vi "daq_board__V3 (2).vi"() -> ()   [LabVIEW 2014]
uses:
  <vilib>/express/express arith-compare/Formula/XNode/ExpressFormulaBlockNode.xnode
  <vilib>/express/express shared/transition.llb/Dynamic To Waveform Array.vi
  <vilib>/express/express arith-compare/Formula/Block/exnFormulaBlock how many pts in the wave.vi
  <vilib>/express/express shared/ex_Modify Signal Name.vi
  <vilib>/express/express shared/transition.llb/Waveform Array To Dynamic.vi
  <vilib>/gmath/NI_Gmath.lvlib
  <vilib>/Utility/file.llb/Write To Spreadsheet File (DBL).vi
  <vilib>/event_ctls.llb/eventsource.ctl
panel:
  out "OK":bool
  in  "Enable":bool=TRUE
  in  "Numeric":i32
  out "Time":u32
  out "true":bool
  in  "stop":bool
  out "time passed (seconds)":i32
  out "Pressure(Torr)":dbl
  out "Voltage(V)":dbl
  out "Waveform Chart 2":dynamicdata(graph)
  out "F-format string":string
  in  "Time to wait(in sec)":dbl
  out "concatenated string":string
  out "Waveform Chart":dbl[](graph)
  in  "stop (F)":bool
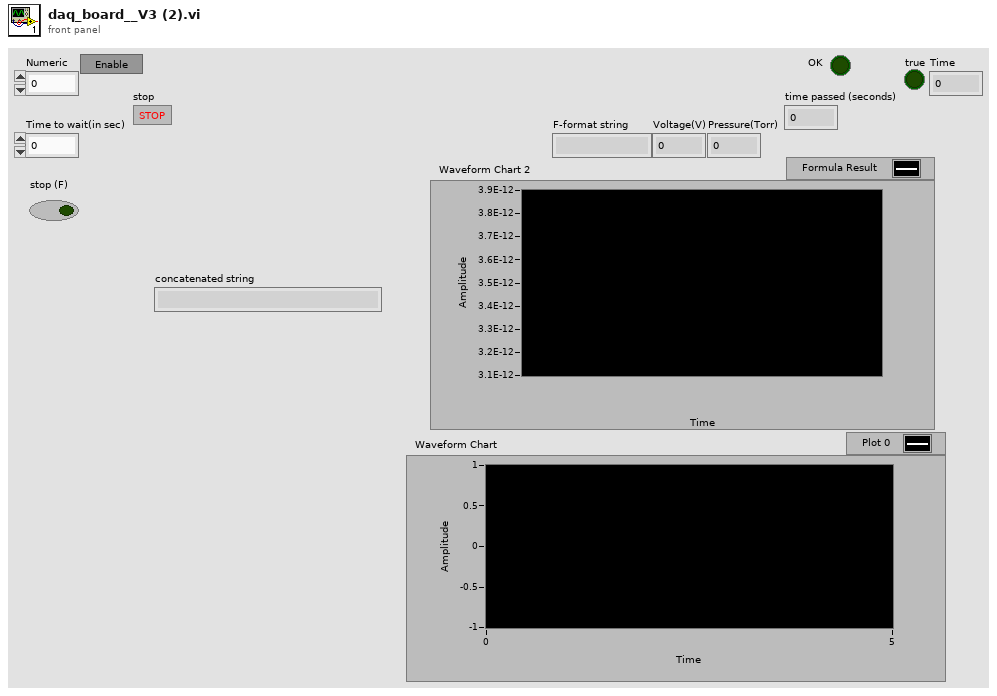
[diagram p1: front panel]
types:
  T1 = typedef "eventsource.ctl" = u32
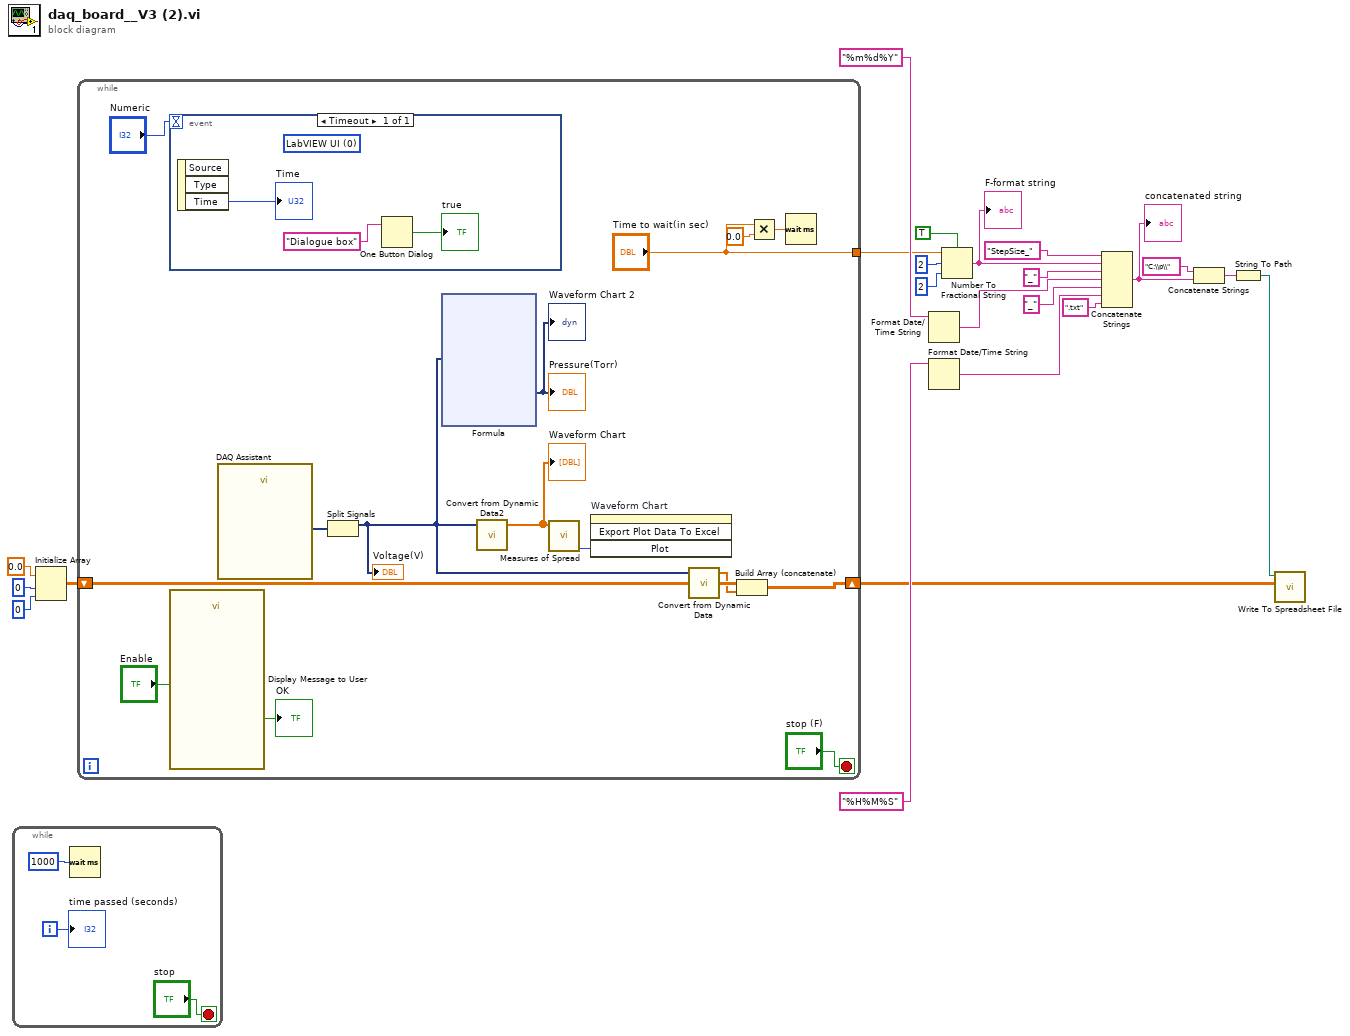
[diagram p0: block diagram]
diagram:
  n1 = while {
    i -> [w25]
    stop <- "stop" stop-if-true
    n2 = Wait (ms)(milliseconds to wait=u32 1000 ("millisecond timer value")) -> ()  [unwired: 1 out]
    "time passed (seconds)" <- w25
  }
  n3 = Initialize Array(0.0 ("Numeric"), 0 ("dimension size"), 0 ("dimension size")) -> (w21:dbl[][])
  n4 = while {
    shift-right: [w37] -> w10
    shift-left: w21 -> [w38]
    tunnel: ["Time to wait(in sec)"] -> w5
    stop <- "stop (F)" stop-if-true
    n5 = event shown="[0] Timeout" {
      selector: _ -> [_]
      dyn-events: _ -> [_]
      timeout: "Numeric" -> [_]
      event Timeout {
        (unwired) T1 0 items=["LabVIEW UI"=0, "ActiveX"=1, "User Event"=25] ("Source")
        n6 = event-data() -> ("Time"=→"Time":u32)  [unwired: 1 in, 2 out]
        n7 = One Button Dialog(message="Dialogue box") -> (true=→"true":bool)  [unwired: 1 in]
      }
    }
    n8 = call "Display Message to User"("Enable"="Enable") -> ("OK"=→"OK":bool)  [unwired: 9 in, 1 out]
    n9 = call "DAQ Assistant"() -> ("data"=w40:dynamicdata)  [unwired: 17 in, 2 out]
    n10 = Split Signals(w40) -> (w28:dynamicdata)  [unwired: 2 in, 1 out]
    "Voltage(V)" <- w28
    n11 = xnode "Formula"("X1"=w28) -> ("Result"=→"Waveform Chart 2" →"Pressure(Torr)":dynamicdata)  [unwired: 1 in, 1 out]
    n12 = call "Convert from Dynamic Data2"("Dynamic Data Type"=w28) -> ("Array"=w30:dbl[])  [unwired: 3 in]
    "Waveform Chart" <- w30
    n13 = call <vilib>:"Measures of Spread.vi"("x array"=w30) -> ("error"=w31:i32)  [unwired: 9 in, 1 out]
    n14 = invoke on="Waveform Chart" class="WFChart (strict)" method="Export Plot Data To Excel"("Plot"=w31) -> ()  [unwired: 3 in, 4 out]
    n15 = call "Convert from Dynamic Data"("Dynamic Data Type"=w28) -> ("Array"=w36:dbl[])  [unwired: 3 in]
    n16 = Build Array (concatenate)(w38, w36) -> (w37:dbl[][])
    n17 = Multiply(x="Time to wait(in sec)", y=0.0) -> (x*y=w35:dbl)
    n18 = Wait (ms)(milliseconds to wait=w35) -> ()  [unwired: 1 out]
  }
  n19 = Format Date/Time String(time format string (%c)="%m%d%Y") -> (date/time string=w16:string)  [unwired: 2 in]
  n20 = Format Date/Time String(time format string (%c)="%H%M%S") -> (date/time string=w14:string)  [unwired: 2 in]
  n21 = Number To Fractional String(use system decimal point (T)=TRUE, number=w5, width (-)=i16 2, precision (6)=i16 2) -> (F-format string=w1:string)
  "F-format string" <- w1
  n22 = Concatenate Strings("StepSize_" ("string"), w1, "_" ("string"), w16, "_" ("string"), w14, ".txt" ("string")) -> (w7:string)
  "concatenated string" <- w7
  n23 = Concatenate Strings("C:\\p\\" ("string"), w7) -> (w6:string)
  n24 = String To Path(string=w6) -> (path=w9:path)
  n25 = call-poly <vilib>:"Write To Spreadsheet File.vi"("2D data"=w10, "file path (dialog if empty)"=w9) -> ()  [unwired: 6 in, 1 out]
